vi "Get_WT_Speed.vi"(1 "Opto Trace":dbl[](array[numeric]) format="%.2f") -> (0 "Samples per pulse":i32[](array[numeric]))   [LabVIEW 2010]
panel:
  out "Waveform Graph":i32[](graph)
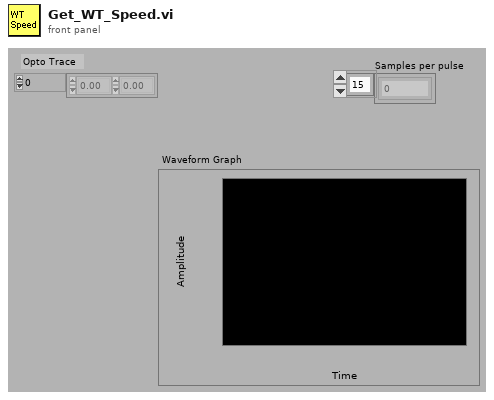
[diagram p1: front panel]
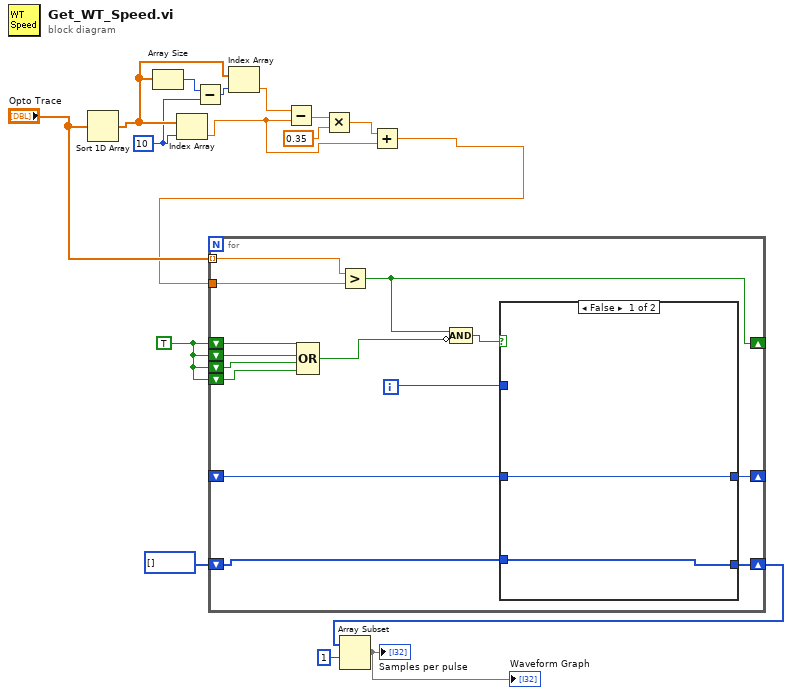
[diagram p0: block diagram]
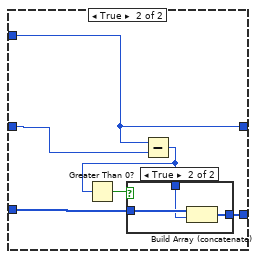
[diagram p2: hidden frame]
diagram:
  w10 = TRUE
  w14 = 10 ("index")
  n1 = Sort 1D Array(array="Opto Trace") -> (sorted array=w16:dbl[])
  n2 = Array Size(array=w16) -> (size(s)=w13:i32)
  n3 = Index Array(array=w16, index=w14) -> (element=w2:dbl)
  n4 = Subtract(x=w13, y=w14) -> (x-y=w15:i32)
  n5 = Index Array(array=w16, index=w15) -> (element=w6:dbl)
  n6 = Subtract(x=w6, y=w2) -> (x-y=w5:dbl)
  n7 = Multiply(x=w5, y=0.35) -> (x*y=w3:dbl)
  n8 = Add(x=w3, y=w2) -> (x+y=w1:dbl)
  n9 = for {
    shift-right: [w17] -> _
    shift-left: w10 -> [w22]
    shift-right: [w27] -> _
    shift-left: _ -> [w26]
    tunnel: "Opto Trace" -> [w30] mode=indexing
    tunnel: w1 -> [w29]
    shift-right: [w24] -> w11
    shift-left: i32[] [] -> [w25]
    shift-left: w10 -> [w21]
    shift-left: w10 -> [w20]
    shift-left: w10 -> [w18]
    i -> [w23]
    n10 = Compound Arithmetic op=OR(w22, w21, w20, w18) -> (w19:bool)
    n11 = Greater?(x=w30, y=w29) -> (0:w17:bool)
    n12 = Compound Arithmetic op=AND(w17, invert w19) -> (w28:bool)
    n13 = case shown="False" w28 {
      tunnel: [w32 w36] -> w27
      tunnel: w23 -> [_ w36]
      tunnel: w26 -> [w32 w35]
      tunnel: w25 -> [w31 w38]
      tunnel: [w31 w37] -> w24
      frame False {
      }
      frame True {
        n14 = Subtract(x=w36, y=w35) -> (x-y=w33:i32)
        n15 = Greater Than 0?(x=w33) -> (x > 0?=w34:bool)
        n16 = case shown="True" w34 {
          tunnel: w38 -> [w39 w42]
          tunnel: [w39 w41] -> w37
          tunnel: w33 -> [_ w40]
          frame False {
          }
          frame True {
            n17 = Build Array (concatenate)(w42, w40) -> (w41:i32[])
          }
        }
      }
    }
  }
  n18 = Array Subset(array=w11, index=1) -> (→"Samples per pulse" →"Waveform Graph":i32[])  [unwired: 1 in]
